vi "CtrlTrain_Analog_Transfer.vi"(4 "Rate 2":dbl, 6 "Rate 1":dbl, 9 "Select 2":bool, 10 "Input 2":dbl, 11 "Input 1":dbl) -> (2 "Output":dbl)   [LabVIEW 2019, in "CtrlTrainingLibary_Protected.lvlib"]
doc: "This VI averages the last seven samples of an analog value. The sample rate is determined by how often this VI is called."
uses:
  CtrlTrainingLibary_Protected.lvlib
  <vilib>/Rock Robotics/WPI/ThirdParty/JAS_Junk/TrajLib/Trajectory_Library.lvlib
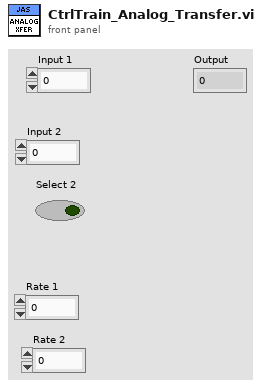
[diagram p1: front panel]
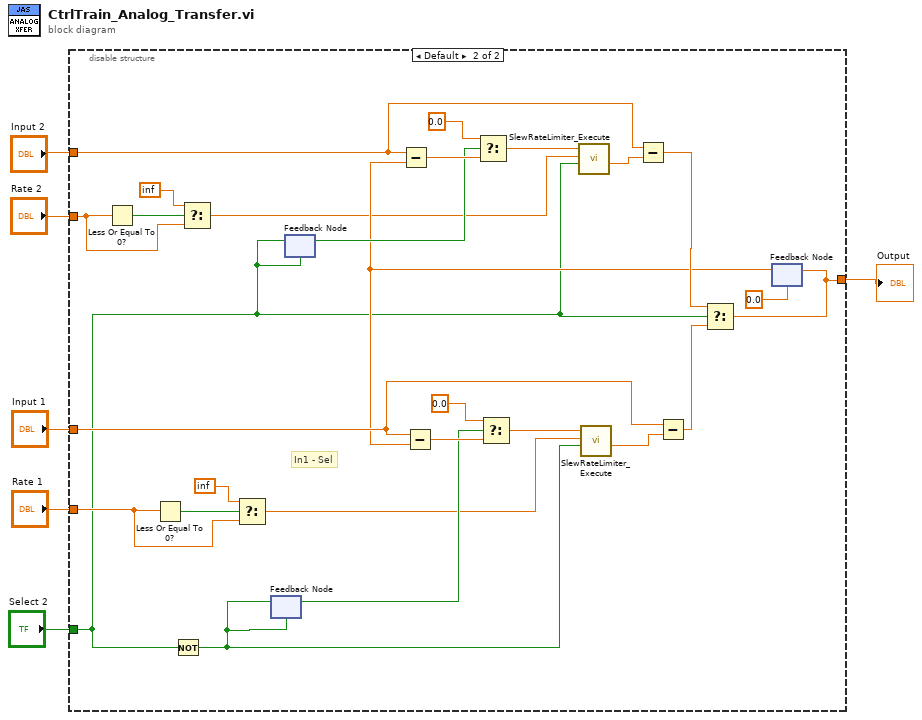
[diagram p0: block diagram]
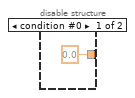
[diagram p2: hidden frame]
diagram:
  n1 = disable-structure shown="Default" {
    disable-tunnel: "Rate 1" -> [_ w32]
    disable-tunnel: "Rate 2" -> [_ w29]
    disable-tunnel: "Input 2" -> [_ w22]
    disable-tunnel: "Input 1" -> [_ w21]
    disable-tunnel: [0.0 w19] -> w2
    disable-tunnel: "Select 2" -> [_ w12]
    frame condition #0 {
    }
    frame condition #1 (active) {
      # "In1 - Sel"
      n2 = Less Or Equal To 0?(x=w29) -> (x <= 0?=w30:bool)
      n3 = Less Or Equal To 0?(x=w32) -> (x <= 0?=w33:bool)
      n4 = Not(x=w12) -> (.not. x?=w10:bool)
      n5 = Select(t=inf, s=w30, f=w29) -> (s? t:f=w13:dbl)
      n6 = Select(t=inf, s=w33, f=w32) -> (s? t:f=w11:dbl)
      n7 = feedback #1(w10) -> (w23:bool)
      n8 = feedback-in #1(w10) -> ()
      n9 = feedback #2(w12) -> (w26:bool)
      n10 = feedback-in #2(w12) -> ()
      n11 = feedback #3(0.0) -> (w17:dbl)
      n12 = Subtract(x=w22, y=w17) -> (x-y=w28:dbl)
      n13 = Subtract(x=w21, y=w17) -> (x-y=w24:dbl)
      n14 = Select(t=0.0, s=w26, f=w28) -> (s? t:f=w15:dbl)
      n15 = Select(t=0.0, s=w23, f=w24) -> (s? t:f=w14:dbl)
      n16 = call <vilib>:"SlewRateLimiter_Execute.vi"("Enable"=w12, "Rate"=w13, "Input"=w15) -> ("Output"=w8:dbl)  [unwired: 7 in, 1 out]
      n17 = call <vilib>:"SlewRateLimiter_Execute.vi"("Enable"=w10, "Rate"=w11, "Input"=w14) -> ("Output"=w9:dbl)  [unwired: 7 in, 1 out]
      n18 = Subtract(x=w22, y=w8) -> (x-y=w18:dbl)
      n19 = Subtract(x=w21, y=w9) -> (x-y=w20:dbl)
      n20 = Select(t=w18, s=w12, f=w20) -> (s? t:f=w19:dbl)
      n21 = feedback-in #3(w19) -> ()
    }
  }
  "Output" <- w2
